vi "2Gear.vi"(9 "2 Gear Side":enum16{"Left", "Right"}(ring), 10 "Gear Side":enum16{"Center", "Left", "Right"}(ring), 11 "RobotDriveDevRef":T1={"DevStatus"={"status"=FALSE, "code"=0, "source"=""}, "Motors[]"=[], "Square Inputs"=FALSE, "Max Output"=1.0}) -> (3 "RobotDriveDevRef 2":T1={"DevStatus"={"status"=FALSE, "code"=0, "source"=""}, "Motors[]"=[], "Square Inputs"=FALSE, "Max Output"=1.0})   [LabVIEW 2016]
uses:
  <vilib>/Rock Robotics/WPI/RobotDrive/WPI_RobotDriveDevRef.ctl
  <vilib>/Rock Robotics/WPI/MotorControl/WPI_MotorControlDeviceRef.ctl
  <vilib>/Rock Robotics/WPI/MotorControl/WPI_MotorControlType.ctl
  <vilib>/Rock Robotics/SystemInterfaces/DIO/FPGA_DIOPWMChannel.ctl
  <vilib>/Rock Robotics/WPI/PWM/WPI_PWMDeadband.ctl
  <vilib>/Rock Robotics/WPI/RobotDrive/WPI_RobotDriveArcadeDrive_Standard(NoSaturation).vi
  Robot Global Data.vi
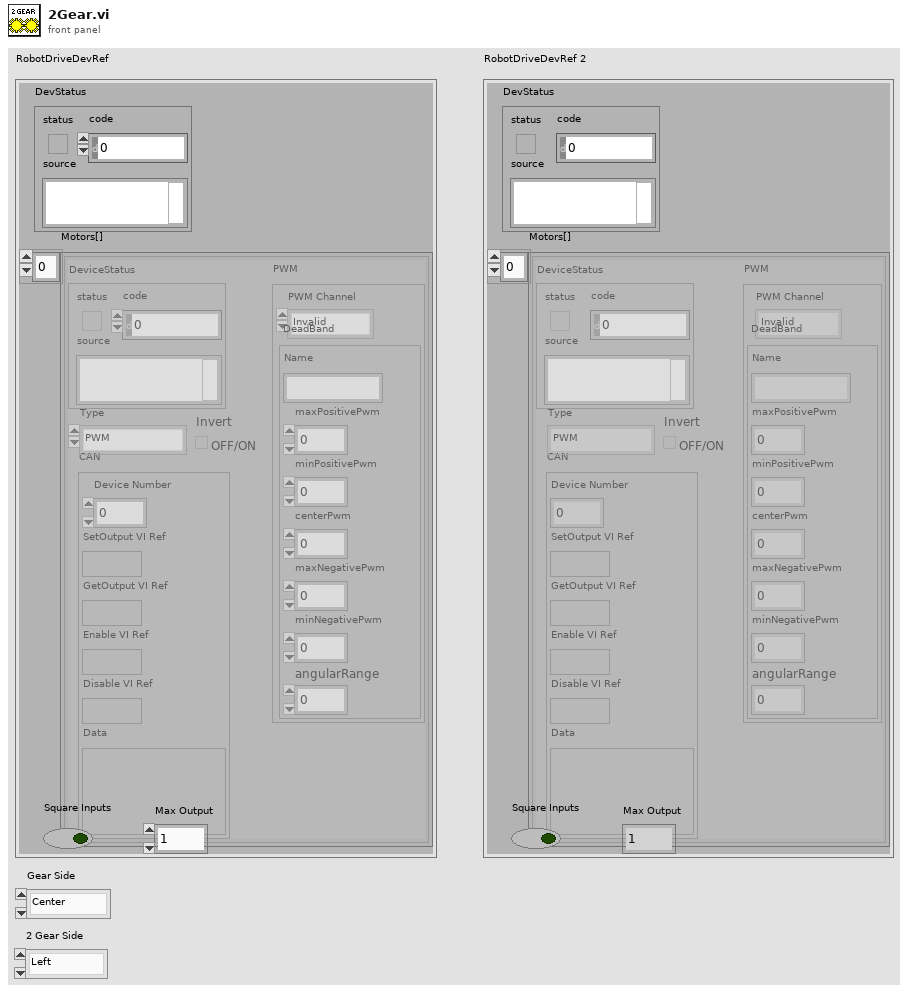
[diagram p1: front panel]
types:
  T1 = typedef "WPI_RobotDriveDevRef.ctl" = cluster{"DevStatus":errorcluster, "Motors[]":T2[], "Square Inputs":bool, "Max Output":dbl}
  T2 = typedef "WPI_MotorControlDeviceRef.ctl" = cluster{"DeviceStatus":errorcluster, "Type":T3, "PWM":cluster{"PWM Channel":T4, "DeadBand":T5}, "CAN":cluster{"Device Number":u8, "SetOutput VI Ref":variant, "GetOutput VI Ref":variant, "Enable VI Ref":variant, "Disable VI Ref":variant, "Data":variant}, "Invert":bool}
  T3 = typedef "WPI_MotorControlType.ctl" = enum16{"PWM", "CAN"}
  T4 = typedef "FPGA_DIOPWMChannel.ctl" = enum8{"PWM 0", "PWM 1", "PWM 2", "PWM 3", "PWM 4", "PWM 5", "PWM 6", "PWM 7", "PWM 8", "PWM 9", "PWM MXP 0", "PWM MXP 1", "PWM MXP 2", "PWM MXP 3", "PWM MXP 4", "PWM MXP 5", "PWM MXP 6", "PWM MXP 7", "PWM MXP 8", "PWM MXP 9", "Invalid"}
  T5 = typedef "WPI_PWMDeadband.ctl" = cluster{"Name":string, "maxPositivePwm":i32, "minPositivePwm":i32, "centerPwm":i32, "maxNegativePwm":i32, "minNegativePwm":i32, "angularRange":u16}
  T6 = cluster{"Target?":bool, "PegAngle":dbl, "Distance":dbl}
  T7 = cluster{"Lower X":dbl, "Lower Y":dbl, "Upper X":dbl, "Upper Y":dbl, "Lower Limit":dbl, "Upper Limit":dbl}
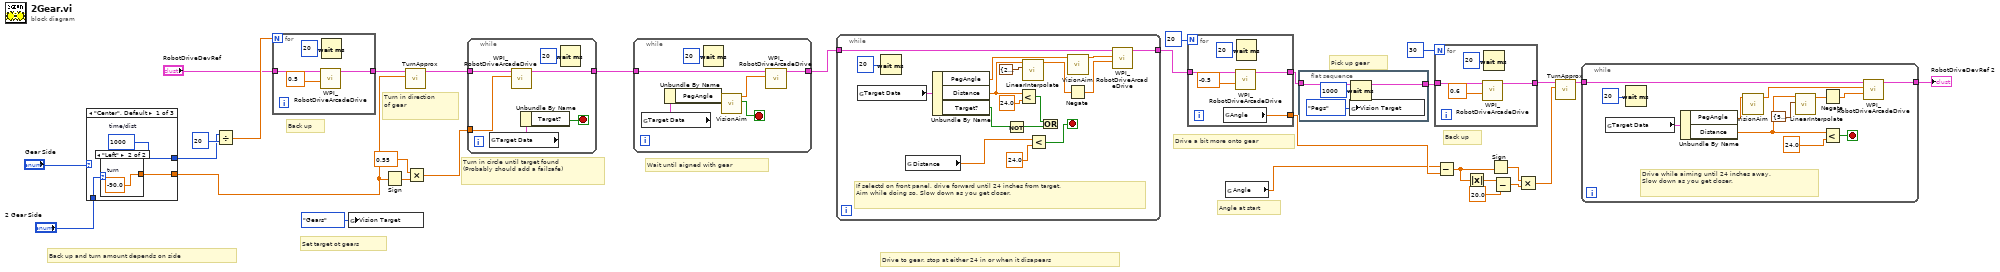
[diagram p0: block diagram]
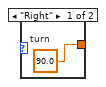
[diagram p2: hidden frame]
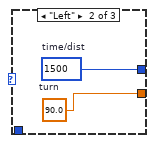
[diagram p3: hidden frame]
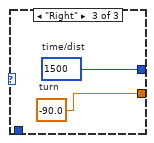
[diagram p4: hidden frame]
diagram:
  # "Set target ot gears"
  # "Angle at start"
  # "Back up"
  # "Pick up gear"
  # "Drive a bit more onto gear"
  # "Drive to gear, stop at either 24 in or when it disapears"
  # "Wait until aigned with gear"
  # "Turn in circle until target found\n(Probably should add a failsafe)"
  # "Turn in direction\nof gear"
  # "Back up"
  # "Back up and turn amount depends on side"
  n1 = case shown="\"Center\", Default" "Gear Side" {
    tunnel: [w33 w37 w39] -> w4
    tunnel: [w34 w38 w40] -> w7
    tunnel: "2 Gear Side" -> [w32 _ _]
    frame "Center", Default {
      w34 = 1000  # time/dist
      n2 = case shown="\"Left\"" w32 {
        tunnel: [w35 w36] -> w33
        frame "Right" {
          w35 = 90.0  # turn
        }
        frame "Left" {
          w36 = -90.0  # turn
        }
      }
    }
    frame "Left" {
      w37 = 90.0  # turn
      w38 = 1500  # time/dist
    }
    frame "Right" {
      w39 = -90.0  # turn
      w40 = 1500  # time/dist
    }
  }
  n3 = Divide(x=w7, y=20) -> (x/y=w29:dbl)
  n4 = for {
    N: w29 -> [_]
    tunnel: "RobotDriveDevRef" -> [w44]
    tunnel: [w42] -> w23
    n5 = call-poly <vilib>:"WPI_RobotDriveArcadeDrive.vi"("Y axis value"=0.5 ("X axis value"), "RobotDriveDevRef"=w44) -> ("RobotDriveDevRef"=w42:T1)  [unwired: 7 in, 2 out]
    n6 = Wait (ms)(milliseconds to wait=u32 20) -> ()  [unwired: 1 out]
  }
  n7 = global write "Robot Global Data.vi" "Vision Target"(enum16{"Pegs", "Gears"}."Gears" ("Vision Target")) -> ()
  n8 = Sign(1:w4) -> (0:w3:dbl)
  n9 = call "TurnApprox.vi"("Angle"=w4, "RobotDriveDevRef"=w23) -> ("RobotDriveDevRef"=w22:T1)  [unwired: 9 in]
  n10 = Multiply(x=0.55 ("X axis value"), y=w3) -> (x*y=w1:dbl)
  n11 = while {
    tunnel: w22 -> [w50]
    tunnel: [w49] -> w27
    tunnel: w1 -> [w45]
    stop <- w46 stop-if-true
    n12 = global read "Robot Global Data.vi" "Target Data"() -> (w47:T6)
    n13 = call-poly <vilib>:"WPI_RobotDriveArcadeDrive.vi"("X axis value"=w45, "RobotDriveDevRef"=w50) -> ("RobotDriveDevRef"=w49:T1)  [unwired: 7 in, 2 out]
    n14 = Unbundle By Name(w47) -> ("Target?"=w46:bool)
    n15 = Wait (ms)(milliseconds to wait=u32 20) -> ()  [unwired: 1 out]
  }
  n16 = while {
    tunnel: w27 -> [w57]
    tunnel: [w53] -> w26
    stop <- w55 stop-if-true
    n17 = global read "Robot Global Data.vi" "Target Data"() -> (w52:T6)
    n18 = Unbundle By Name(w52) -> ("PegAngle"=w51:dbl)
    n19 = Wait (ms)(milliseconds to wait=u32 20) -> ()  [unwired: 1 out]
    n20 = call "VisionAim.vi"("Angle"=w51) -> ("In Range"=w55:bool, "Turn Amount"=w56:dbl)  [unwired: 9 in]
    n21 = call-poly <vilib>:"WPI_RobotDriveArcadeDrive.vi"("X axis value"=w56, "RobotDriveDevRef"=w57) -> ("RobotDriveDevRef"=w53:T1)  [unwired: 7 in, 2 out]
  }
  n22 = while {
    tunnel: w26 -> [w73]
    tunnel: [w72] -> w25
    stop <- w58 stop-if-true
    # "If selectd on front panel, drive forward until 24 inches from target.\nAim while doing so. Slow down as you get closer."
    n23 = global read "Robot Global Data.vi" "Target Data"() -> (w68:T6)
    n24 = Wait (ms)(milliseconds to wait=u32 20) -> ()  [unwired: 1 out]
    n25 = global read "Robot Global Data.vi" "Distance"() -> (w60:dbl)
    n26 = Unbundle By Name(w68) -> ("PegAngle"=w67:dbl, "Distance"=w62:dbl, "Target?"=w64:bool)
    n27 = Not(x=w64) -> (.not. x?=w65:bool)
    n28 = Less?(x=w62, y=24.0) -> (x < y?=w66:bool)
    n29 = call "LinearInterpolate.vi"("Config"=T7 {"Lower X"=24.0, "Lower Y"=0.48, "Upper X"=65.0, "Upper Y"=0.8, "Lower Limit"=0.45, "Upper Limit"=0.75}, "Value"=w62) -> ("Ouput"=w61:dbl)  [unwired: 9 in]
    n30 = Less?(x=w60, y=24.0) -> (x < y?=w58:bool)
    n31 = Or(x=w66, y=w65) -> ()  [unwired: 1 out]
    n32 = Negate(x=w61) -> (-x=w69:dbl)
    n33 = call "VisionAim.vi"("Angle"=w67) -> ("Turn Amount"=w74:dbl)  [unwired: 9 in, 1 out]
    n34 = call-poly <vilib>:"WPI_RobotDriveArcadeDrive.vi"("Y axis value"=w69, "X axis value"=w74, "RobotDriveDevRef"=w73) -> ("RobotDriveDevRef"=w72:T1)  [unwired: 6 in, 2 out]
  }
  n35 = for {
    N: 20 -> [_]
    tunnel: w25 -> [w79]
    tunnel: [w77] -> w18
    tunnel: [w75] -> w19
    n36 = global read "Robot Global Data.vi" "Angle"() -> (w75:dbl)
    n37 = call-poly <vilib>:"WPI_RobotDriveArcadeDrive.vi"("Y axis value"=-0.5 ("X axis value"), "RobotDriveDevRef"=w79) -> ("RobotDriveDevRef"=w77:T1)  [unwired: 7 in, 2 out]
    n38 = Wait (ms)(milliseconds to wait=u32 20) -> ()  [unwired: 1 out]
  }
  n39 = global read "Robot Global Data.vi" "Angle"() -> (w16:dbl)
  n40 = flat-sequence {
    tunnel: w18 -> [w82]
    tunnel: [w82] -> w17
    frame #0 {
      n41 = global write "Robot Global Data.vi" "Vision Target"(enum16{"Pegs", "Gears"}."Pegs" ("Vision Target")) -> ()
      n42 = Wait (ms)(milliseconds to wait=u32 1000) -> ()  [unwired: 1 out]
    }
  }
  n43 = for {
    N: 30 -> [_]
    tunnel: w17 -> [w86]
    tunnel: [w84] -> w20
    n44 = call-poly <vilib>:"WPI_RobotDriveArcadeDrive.vi"("Y axis value"=0.6 ("X axis value"), "RobotDriveDevRef"=w86) -> ("RobotDriveDevRef"=w84:T1)  [unwired: 7 in, 2 out]
    n45 = Wait (ms)(milliseconds to wait=u32 20) -> ()  [unwired: 1 out]
  }
  n46 = Subtract(x=w16, y=w19) -> (x-y=w11:dbl)
  n47 = Absolute Value(x=w11) -> (abs(x)=w14:dbl)
  n48 = Sign(1:w11) -> (0:w10:dbl)
  n49 = Subtract(x=w14, y=20.0) -> (x-y=w12:dbl)
  n50 = Multiply(x=w10, y=w12) -> (x*y=w9:dbl)
  n51 = call "TurnApprox.vi"("Angle"=w9, "RobotDriveDevRef"=w20) -> ("RobotDriveDevRef"=w15:T1)  [unwired: 9 in]
  n52 = while {
    tunnel: w15 -> [w98]
    tunnel: [w97] -> w8
    stop <- w95 stop-if-true
    # "Drive while aiming until 24 inches away.\nSlow down as you get closer."
    n53 = global read "Robot Global Data.vi" "Target Data"() -> (w92:T6)
    n54 = Wait (ms)(milliseconds to wait=u32 20) -> ()  [unwired: 1 out]
    n55 = Unbundle By Name(w92) -> ("PegAngle"=w91:dbl, "Distance"=w87:dbl)
    n56 = call "VisionAim.vi"("Angle"=w91) -> ("Turn Amount"=w89:dbl)  [unwired: 9 in, 1 out]
    n57 = call "LinearInterpolate.vi"("Config"=T7 {"Lower X"=55.0, "Lower Y"=0.48, "Upper X"=65.0, "Upper Y"=0.8, "Lower Limit"=0.45, "Upper Limit"=0.75}, "Value"=w87) -> ("Ouput"=w88:dbl)  [unwired: 9 in]
    n58 = Negate(x=w88) -> (-x=w93:dbl)
    n59 = Less?(x=w87, y=24.0) -> (x < y?=w95:bool)
    n60 = call-poly <vilib>:"WPI_RobotDriveArcadeDrive.vi"("Y axis value"=w93, "X axis value"=w89, "RobotDriveDevRef"=w98) -> ("RobotDriveDevRef"=w97:T1)  [unwired: 6 in, 2 out]
  }
  "RobotDriveDevRef 2" <- w8
